vi "Gather Test Data - Heatup Test new.vi"(0 "Agilent Scan List":string="101,102,103,104,105,106,107,108,109,110,111,112,113,114,115,116", 1 "Semiphore":T3, 2 "Equipment":T5={"COM Port"="COM1", "MW100"="MW100", "AG34970"="A-34972A", "Chamber"="WT500"}, 5 "Tank Display Ref":refnum<vi>, 7 "Agilent?":bool=TRUE, 9 "Calibration Coefficients":dbl[][](array[numeric]), 11 "error in (no error)":errorcluster, 13 "Serial Data In":string, 14 "Agilent Label Array":string[](array[string])) -> (4 "Tc Tree":dbl[](array[numeric]) format="%.4f", 6 "Output Data":string[][](array[string]), 8 "POWER":T1, 10 "PowerData":T2={"Voltage"=236.2, "Current"=17.749, "Power"=4192.0, "WattHours"=0.0}, 12 "Voltage":dbl=240.0, 15 "error out":errorcluster={"status"=TRUE, "code"=-1073807346, "source"="VISA Read in Gather Test Data.vi"})   [LabVIEW 2012]
uses:
  EquipReferences.ctl
  HEWH Tank Indicator.ctl
  PowerData.ctl
  PowerElements.ctl
panel:
  out "MW100 Raw Data":string[](array[string])
  out "34970 Raw Data":string[](array[string])
  out "Flow(GPM)":dbl
  out "Gallons":dbl
  out "Tambient":dbl
  out "34970 Data":string[](array[string])=["32.000000E+0"]
  out "Local Tank Display":T4 {"TC6" format="%.2g"; "TIN" format="%.2g"; "TOUT" format="%.2g"; "Mean" format="%.2f"; "Std Dev" format="%.2f"; "TC5" format="%.2g"; "TC4" format="%.2g"; "TC3" format="%.2g"; "TC2" format="%.2g"; "TC1" format="%.2g"}
  out "MW100 Data":string[](array[string])=["0.000000E+0", "0.000000E+0"]
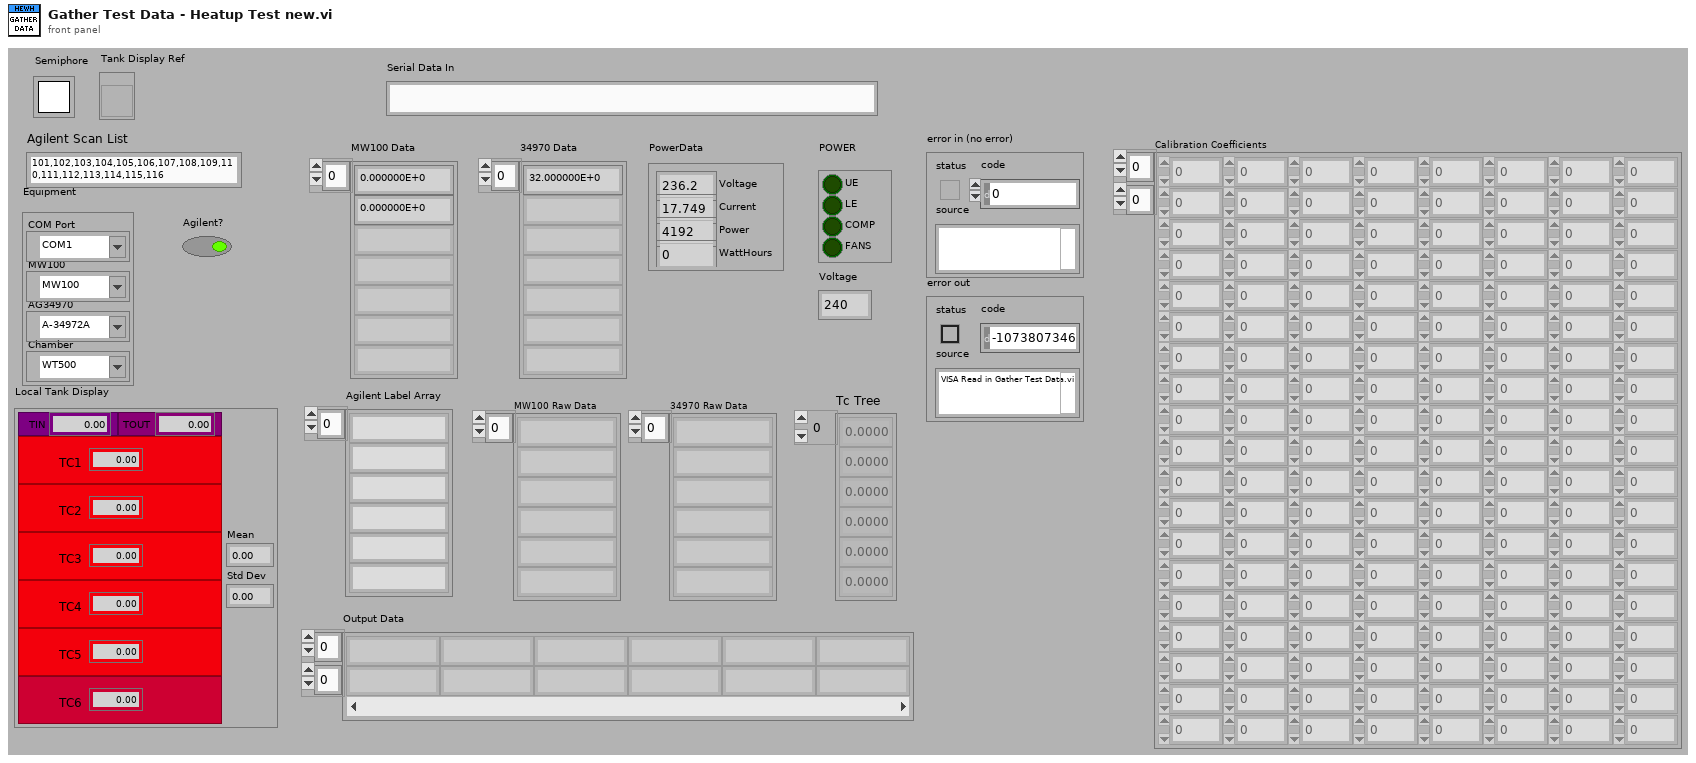
[diagram p1: front panel]
types:
  T1 = typedef "PowerElements.ctl" = cluster{"UE":bool, "LE":bool, "COMP":bool, "FANS":bool}
  T2 = typedef "PowerData.ctl" = cluster{"Voltage":dbl, "Current":dbl, "Power":dbl, "WattHours":dbl}
  T3 = typedef "Semaphore RefNum" = refnum<k1>
  T4 = typedef "HEWH Tank Indicator.ctl" = cluster{"TC1-D":bool, "TC2-D":bool, "TC3-D":bool, "TC4-D":bool, "TC5-D":bool, "RTD_IN":bool, "RTDOUT":bool, "TC1":dbl, "TC2":dbl, "TC3":dbl, "TC4":dbl, "TC5":dbl, "TIN":dbl, "TOUT":dbl, "Std Dev":dbl, "Mean":dbl, "TC6-D":bool, "TC6":dbl}
  T5 = typedef "EquipReferences.ctl" = cluster{"COM Port":refnum<visa-resource-name>, "MW100":refnum<visa-resource-name>, "AG34970":refnum<visa-resource-name>, "Chamber":refnum<visa-resource-name>}
  T6 = typedef "PowerClassification.ctl" = cluster{"Off":bool, "On":bool, "Fans":bool, "Compressor":bool, "Heat Elem.":bool, "Fault-OverPwr":bool}
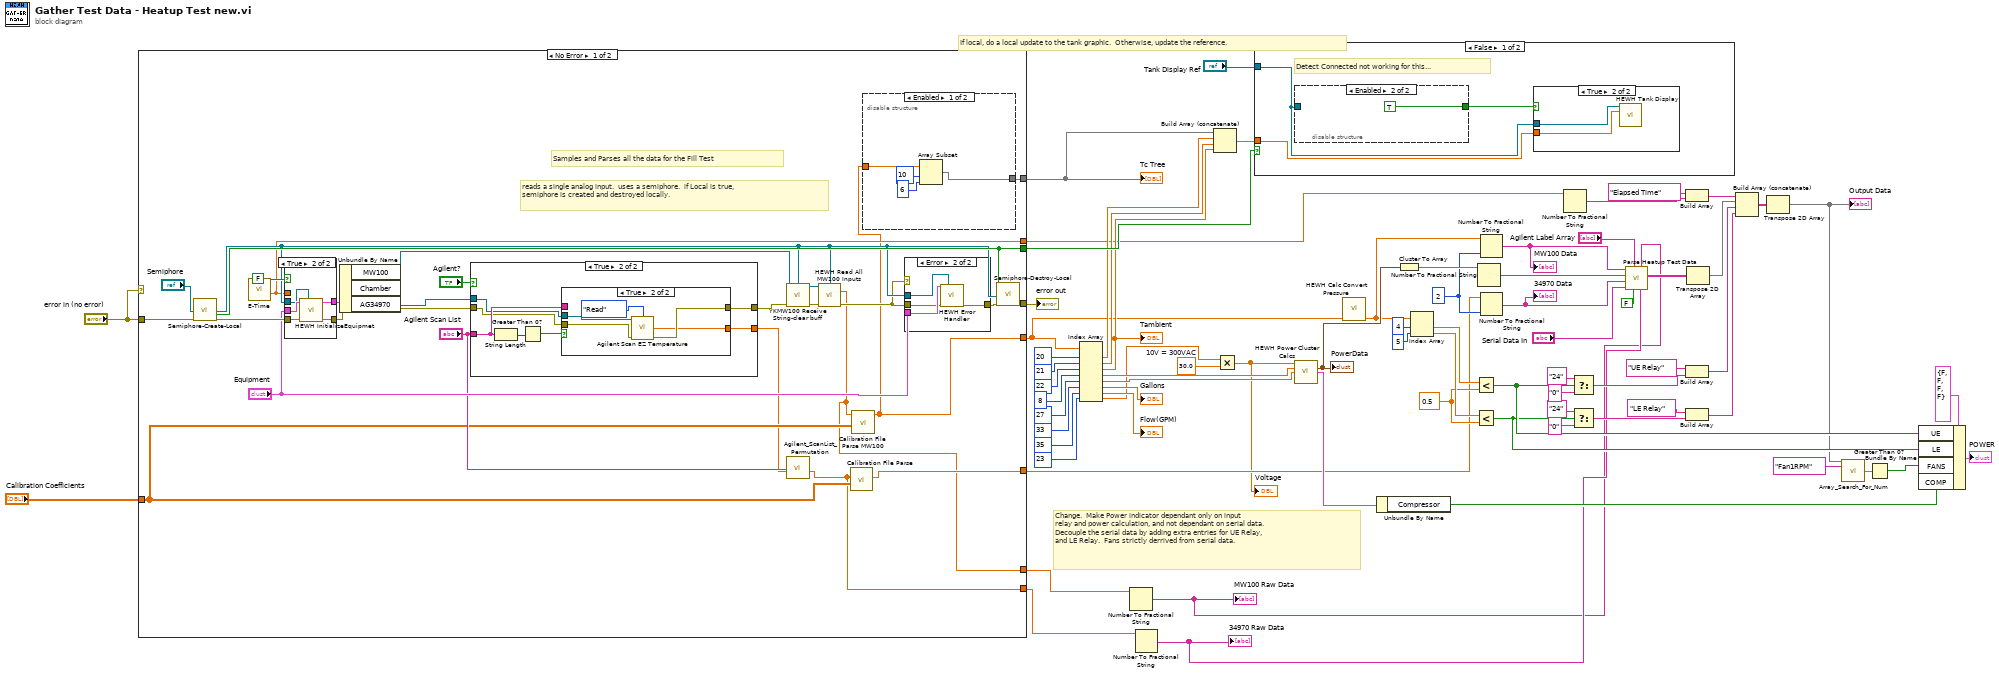
[diagram p0: block diagram]
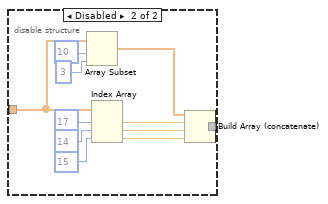
[diagram p2: hidden frame]
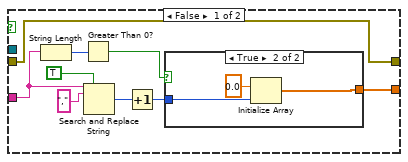
[diagram p3: hidden frame]
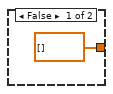
[diagram p4: hidden frame]
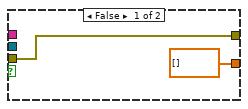
[diagram p5: hidden frame]
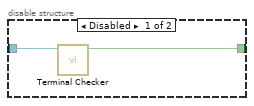
[diagram p9: hidden frame]
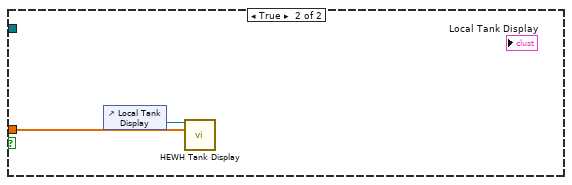
[diagram p11: hidden frame]
diagram:
  w21 = 30.0  # 10V = 300VAC
  w28 = 0.5 ("y")
  w47 = i16 2 ("precision (6)")
  # "Change.  Make Power indicator dependant only on input\nrelay and power calculation, and not dependant on serial data.\nDecouple the serial data by adding extra entries for UE Relay,\nand LE Relay.  Fans strictly derrived from serial data."
  # "If local, do a local update to the tank graphic.  Otherwise, update the reference."
  n1 = case shown="No Error" "error in (no error)" {
    tunnel: "error in (no error)" -> [w99 w155]
    tunnel: [w94 _] -> w66
    tunnel: [w92 w155] -> w65
    tunnel: [w88 _] -> w63
    tunnel: [w78 _] -> w46
    tunnel: [w80 _] -> w44
    tunnel: [w79 _] -> w27
    tunnel: "Calibration Coefficients" -> [w77 _]
    tunnel: [w74 _] -> w3
    tunnel: [w75 _] -> w4
    frame No Error {
      # "reads a single analog input.  uses a semiphore.  if Local is true, \nsemiphore is created and destroyed locally."
      # "Samples and Parses all the data for the Fill Test"
      n2 = call "Semiphore-Create-Local.vi"("Semiphore"="Semiphore", "error in (no error)"=w99) -> ("semaphore"=w87:T3, "Local?"=w94:bool, "error out"=w97:errorcluster)  [unwired: 15 in]
      n3 = call "E-Time.vi"() -> ("Elapsed Time (sec)"=w80:dbl)  [unwired: 9 in, 2 out]
      n4 = case shown="True" FALSE ("No Serial?") {
        tunnel: [w149 w153] -> w98
        tunnel: "Equipment" -> [w149 w154]
        tunnel: w97 -> [w148 w152]
        tunnel: [w148 w151] -> w81
        tunnel: w87 -> [_ w150]
        tunnel: w80 -> [_ _]
        frame False {
        }
        frame True {
          n5 = call "HEWH InitializeEquipmet.vi"("Semiphore"=w150, "Error In"=w152, "Equipment"=w154) -> ("Error Out"=w151:errorcluster, "Equipment Out"=w153:T5)  [unwired: 5 in, 2 out]
        }
      }
      n6 = Unbundle By Name(w98) -> ("MW100"=w91:refnum<visa-resource-name>, "AG34970"=w85:refnum<visa-resource-name>)  [unwired: 1 out]
      n7 = case shown="True" "Agilent?" {
        tunnel: [w117 w133] -> w76
        tunnel: w85 -> [_ w131]
        tunnel: "Agilent Scan List" -> [w121 w132]
        tunnel: w81 -> [w124 w130]
        tunnel: [w124 w129] -> w84
        frame False {
          n8 = String Length(string=w121) -> (length=w120:i32)
          n9 = Greater Than 0?(x=w120) -> (x > 0?=w119:bool)
          n10 = Search and Replace String(replace all?=TRUE ("ignore case? (F)"), input string=w121, search string=",") -> (number of replacements=w122:i32)  [unwired: 5 in, 3 out]
          n11 = Increment(x=w122) -> (x+1=w118:i32)
          n12 = case shown="True" w119 {
            tunnel: w118 -> [_ w127]
            tunnel: [dbl[] [] w126] -> w117
            frame False {
            }
            frame True {
              n13 = Initialize Array(0.0, w127) -> (w126:dbl[])
            }
          }
        }
        frame True {
          n14 = String Length(string=w132) -> (length=w135:i32)
          n15 = Greater Than 0?(x=w135) -> (x > 0?=w134:bool)
          n16 = case shown="True" w134 {
            tunnel: [dbl[] [] w139] -> w133
            tunnel: w132 -> [_ _]
            tunnel: w131 -> [_ w142]
            tunnel: w130 -> [w136 w141]
            tunnel: [w136 w140] -> w129
            frame False {
            }
            frame True {
              n17 = call "Agilent Scan EZ Temperature.vi"("VISA Resource Name"=w142, "Control"=enum16{"Initialize", "Read", "Experiment"}."Read", "error in (no error)"=w141) -> ("Output Array"=w139:dbl[], "error out"=w140:errorcluster)  [unwired: 9 in, 2 out]
            }
          }
        }
      }
      n18 = call "YKMW100 Receive String-clear buff.vi"("VISA session"=w91, "Semiphore"=w87, "error in (no error)"=w84) -> ("dup VISA session"=w90:refnum<visa-resource-name>, "error out"=w89:errorcluster)  [unwired: 10 in, 1 out]
      n19 = call "Agilent_ScanList_Permutation.vi"("Input Data Array"=w76, "Agilent Scan List"="Agilent Scan List") -> ("Output Data Permutation"=w74:dbl[])  [unwired: 9 in]
      n20 = call "HEWH Read All MW100 Inputs.vi"("MW100"=w90, "Semiphore"=w87, "Error In"=w89) -> ("All Data"=w75:dbl[], "error out"=w82:errorcluster)  [unwired: 10 in, 1 out]
      n21 = call "Calibration File Parse.vi"("Calibration Coefficients"=w77, "34972 Array"=w74) -> ("34972 Calibration"=w79:dbl[])  [unwired: 6 in, 1 out]
      n22 = call "Calibration File Parse MW100.vi"("Calibration Coefficients"=w77, "MW100 Array"=w75) -> ("MW100 Calibration"=w78:dbl[])  [unwired: 6 in, 1 out]
      n23 = disable-structure shown="Enabled" {
        disable-tunnel: [w102 w109] -> w88
        disable-tunnel: w78 -> [w101 w113]
        frame Enabled {
          n24 = Array Subset(array=w101, index=10, length=6) -> (w102:dbl[])
        }
        frame Disabled {
          n25 = Array Subset(array=w113, index=10, length=3) -> (w105:dbl[])
          n26 = Index Array(array=w113, index #1=17 ("index"), index #2=14 ("index"), index #3=15 ("index")) -> (element #1=w106:dbl, element #2=w107:dbl, element #3=w108:dbl)
          n27 = Build Array (concatenate)(w105, w106, w107, w108) -> (w109:dbl[])
        }
      }
      n28 = case shown="Error" w82 {
        tunnel: "Equipment" -> [_ w147]
        tunnel: [w143 w146] -> w93
        tunnel: w87 -> [_ w145]
        tunnel: w82 -> [w143 w144]
        frame No Error {
        }
        frame Error {
          n29 = call "HEWH Error Handler.vi"("Equipment"=w147, "MW100 Semiphore"=w145, "error in (no error)"=w144) -> ("Error Out (no error)"=w146:errorcluster)  [unwired: 12 in]
        }
      }
      n30 = call "Semiphore-Destroy-Local.vi"("Semiphore"=w87, "Local?"=w94, "error in (no error)"=w93) -> ("error out"=w92:errorcluster)  [unwired: 16 in]
    }
    frame Error {
    }
  }
  "error out" <- w65
  "Tc Tree" <- w63
  n31 = Index Array(array=w46, index #1=20 ("index"), index #2=21 ("index"), index #3=22 ("index"), index #4=8 ("index"), index #5=27 ("index"), index #6=33 ("index"), index #7=35 ("index"), index #8=23 ("index")) -> (element #1=w61:dbl, element #2=w59:dbl, element #3=w57:dbl, element #4=w50:dbl, element #5=w49:dbl, element #6=→"Gallons":dbl, element #7=→"Flow(GPM)":dbl, element #8=w22:dbl)
  "Tambient" <- w57
  n32 = Number To Fractional String(number=w4) -> (F-format string=w1:string[])  [unwired: 3 in]
  "MW100 Raw Data" <- w1
  n33 = Number To Fractional String(number=w3) -> (F-format string=w2:string[])  [unwired: 3 in]
  "34970 Raw Data" <- w2
  n34 = Build Array (concatenate)(w63, w61, w59, w57) -> (w69:dbl[])
  n35 = Multiply(x=w22, y=w21) -> (x*y=w23:dbl)
  "Voltage" <- w23
  n36 = case shown="False" w66 {
    tunnel: w69 -> [w158 w165]
    tunnel: "Tank Display Ref" -> [w156 _]
    frame False {
      # "Detect Connected not working for this..."
      n37 = disable-structure shown="Enabled" {
        disable-tunnel: [w160 TRUE ("is connected?")] -> w157
        disable-tunnel: w156 -> [w159 _]
        frame Disabled {
          n38 = call "Terminal Checker.vi"("control reference"=w159) -> ("is connected?"=w160:bool)  [unwired: 9 in, 1 out]
        }
        frame Enabled {
        }
      }
      n39 = case shown="True" w157 {
        tunnel: w158 -> [_ w163]
        tunnel: w156 -> [_ w162]
        frame False {
        }
        frame True {
          n40 = call "HEWH Tank Display.vi"("Local Tank Display"=w162, "T1-T6.Tin,Tout"=w163) -> ()  [unwired: 13 in, 1 out]
        }
      }
    }
    frame True {
      n41 = control-ref of="Local Tank Display"() -> (w164:refnum<vi>)
      n42 = call "HEWH Tank Display.vi"("Local Tank Display"=w164, "T1-T6.Tin,Tout"=w165) -> ()  [unwired: 13 in, 1 out]
    }
  }
  n43 = call "HEWH Power Cluster Calcs.vi"("Voltage"=w23, "Watts"=w50, "WattHours"=w49) -> ("PowerData"=w48:T2, "PowerClass"=w32:T6)  [unwired: 11 in]
  "PowerData" <- w48
  n44 = call "HEWH Calc Convert Pressure.vi"("All Data"=w46) -> ("output array"=w36:dbl[])  [unwired: 10 in]
  n45 = Unbundle By Name(w32) -> ("Compressor"=w31:bool)
  n46 = Cluster To Array(cluster=w48) -> (array=w72:dbl[])
  n47 = Index Array(array=w36, index #1=4 ("index"), index #2=5 ("index")) -> (element #1=w39:dbl, element #2=w40:dbl)
  n48 = Less?(x=w39, y=w28) -> (x < y?=w30:bool)
  n49 = Less?(x=w40, y=w28) -> (x < y?=w29:bool)
  n50 = Number To Fractional String(number=w72) -> (F-format string=w71:string[])  [unwired: 3 in]
  n51 = Number To Fractional String(number=w36, precision (6)=w47) -> (F-format string=w73:string[])  [unwired: 2 in]
  "MW100 Data" <- w73
  n52 = Number To Fractional String(number=w27, precision (6)=w47) -> (F-format string=w70:string[])  [unwired: 2 in]
  "34970 Data" <- w70
  n53 = Number To Fractional String(number=w44) -> (F-format string=w17:string)  [unwired: 3 in]
  n54 = Select(t="24" ("trimmed string"), s=w30, f="0" ("trimmed string")) -> (s? t:f=w34:string)
  n55 = Select(t="24" ("trimmed string"), s=w29, f="0" ("trimmed string")) -> (s? t:f=w33:string)
  n56 = call "Parse Heatup Test Data.vi"("34970 Data Raw"=w2, "MW100 Data Raw"=w1, "Agilent Read All?"=FALSE, "Agilent Label Array"="Agilent Label Array", "Serial Data"="Serial Data In", "34970 Data"=w70, "Power Data"=w71, "MW100 Data"=w73) -> ("Output Data"=w68:string[][])  [unwired: 3 in]
  n57 = Build Array("Elapsed Time" ("Serial Data 2"), w17) -> (w19:string[])
  n58 = Build Array("UE Relay" ("Serial Data 2"), w34) -> (w13:string[])
  n59 = Build Array("LE Relay" ("Serial Data 2"), w33) -> (w11:string[])
  n60 = Transpose 2D Array(2D array=w68) -> (transposed array=w67:string[][])
  n61 = Build Array (concatenate)(w19, w67, w13, w11) -> (w18:string[][])
  n62 = Transpose 2D Array(2D array=w18) -> (transposed array=w9:string[][])
  "Output Data" <- w9
  n63 = call "Array_Search_For_Num.vi"("N Rows of Data"=w9, "Title?"="Fan1RPM" ("trimmed string")) -> ("number"=w8:dbl)  [unwired: 12 in, 1 out]
  n64 = Greater Than 0?(x=w8) -> (x > 0?=w7:bool)
  n65 = Bundle By Name(cluster=T1 {"UE"=FALSE, "LE"=FALSE, "COMP"=FALSE, "FANS"=FALSE} ("POWER"), "UE"=w30, "LE"=w29, "FANS"=w7, "COMP"=w31) -> (→"POWER":T1)
